vi "MSEncoder Act Init.vi"(6 "error in (no error)":errorcluster, 8 "scriptPythonCode":string, 9 "eventProcess":string[][](array[string])) -> (0 "error out":errorcluster, 3 "MSEncoder out":refnum<class "MSEncoder.lvclass">)   [LabVIEW 2018, in "MSEncoder.lvclass"]
uses:
  MSEncoder.lvclass
  Ctl/MSEditorParam updConj.ctl
  MSEncoder.lvclass/MSEncoder.ctl
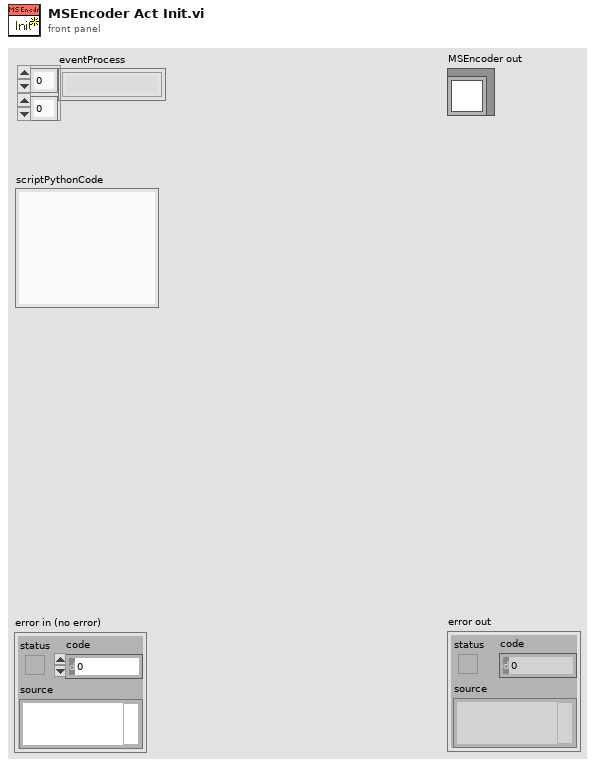
[diagram p1: front panel]
types:
  T1 = typedef "MSEditorParam updConj.ctl" = cluster{"iniPhase":u32, "conjLen":ext[], "phaseDiff":u64[], "fixedLen":bool}
  T2 = cluster{"Freq":ext, "Amp":ext, "Decyc":u32, "1/Decyc":u32, "MaxAmp":dbl}
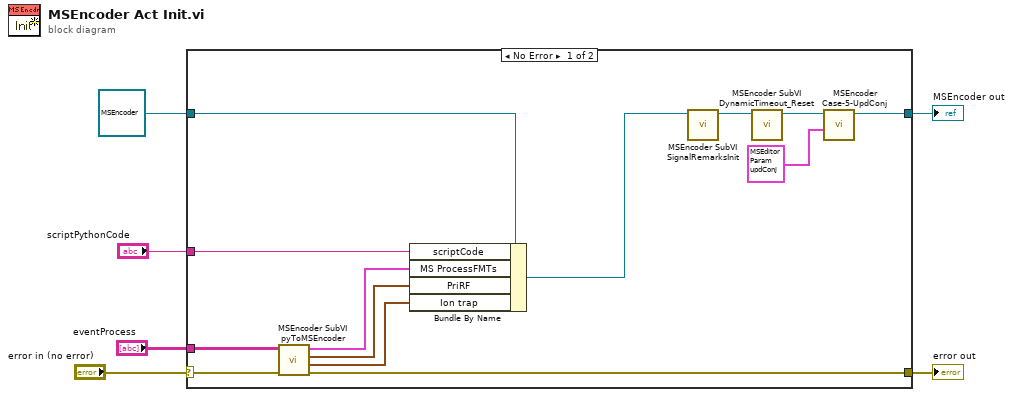
[diagram p0: block diagram]
diagram:
  n1 = case shown="No Error" "error in (no error)" {
    selector: "error in (no error)" -> [w13 w21]
    tunnel: [w12 w21] -> w5
    tunnel: [w15 w20] -> w3
    tunnel: refnum<class "MSEncoder.lvclass"> refnum ("MSEncoder in") -> [w19 w20]
    tunnel: "eventProcess" -> [w7 _]
    tunnel: "scriptPythonCode" -> [w8 _]
    frame No Error {
      n2 = call "MSEncoder SubVI pyToMSEncoder.vi"("error in (no error)"=w13, "eventProcess"=w7) -> ("error out"=w12:errorcluster, "Ion trap"=w9:cluster{"R0":ext, "Z0":ext}, "PriRF"=w10:T2, "MS ProcessFMTs"=w11:cluster{"ProcessName":string, "Data":variant}[])  [unwired: 6 in]
      n3 = Bundle By Name(cluster=w19, "scriptCode"=w8, "MS ProcessFMTs"=w11, "PriRF"=w10, "Ion trap"=w9) -> (w17:refnum<class "MSEncoder.lvclass">)
      n4 = call "MSEncoder SubVI SignalRemarksInit.vi"("MSEncoder in"=w17) -> ("MSEncoder out"=w18:refnum<class "MSEncoder.lvclass">)  [unwired: 10 in]
      n5 = call "MSEncoder SubVI DynamicTimeout_Reset.vi"("MSEncoder in"=w18) -> ("MSEncoder out"=w16:refnum<class "MSEncoder.lvclass">)  [unwired: 9 in, 1 out]
      n6 = call "MSEncoder Case-5-UpdConj.vi"("ParamValIn"=T1 {"iniPhase"=2147483648, "conjLen"=[0.0, 0.0], "phaseDiff"=[2147483648, 2147483648], "fixedLen"=FALSE} ("ParamValueType"), "MSEncoder in"=w16) -> ("MSEncoder out"=w15:refnum<class "MSEncoder.lvclass">)  [unwired: 8 in, 1 out]
    }
    frame Error {
    }
  }
  "error out" <- w5
  "MSEncoder out" <- w3
